vi "Calc Bearing Distance.vi"(10 "Current Location":cluster{"Latitude":ext, "Longitude":ext} {"Longitude" format="%#.6f"; "Latitude" format="%#.6f"}, 11 "Destination":cluster{"Latitude":ext, "Longitude":ext} {"Longitude" format="%#.6f"; "Latitude" format="%#.6f"}) -> (2 "Bearing to Destination":dbl, 3 "distance (m)":dbl)   [LabVIEW 2015, in "RDS Libraries.lvlib"]
uses:
  RDS Libraries.lvlib
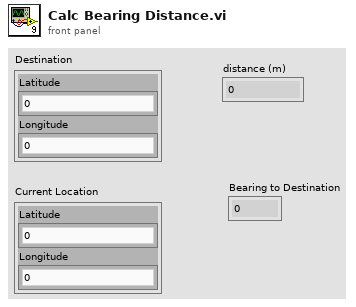
[diagram p1: front panel]
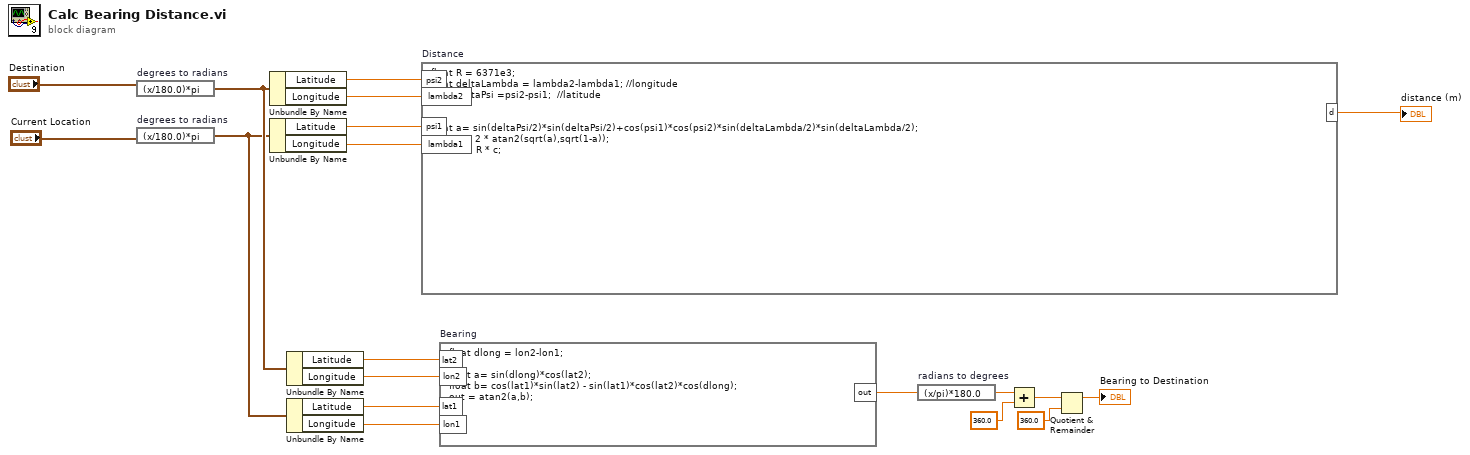
[diagram p0: block diagram]
diagram:
  n1 = expression code="(x/180.0)*pi" "degrees to radians"("Destination") -> (w4:cluster{"Latitude":ext, "Longitude":ext})
  n2 = expression code="(x/180.0)*pi" "degrees to radians"("Current Location") -> (w3:cluster{"Latitude":ext, "Longitude":ext})
  n3 = Unbundle By Name(w4) -> ("Latitude"=w17:ext, "Longitude"=w16:ext)
  n4 = Unbundle By Name(w3) -> ("Latitude"=w19:ext, "Longitude"=w18:ext)
  n5 = Unbundle By Name(w4) -> ("Latitude"=w12:ext, "Longitude"=w11:ext)
  n6 = Unbundle By Name(w3) -> ("Latitude"=w14:ext, "Longitude"=w13:ext)
  n7 = formula code="float R = 6371e3;\nfloat deltaLambda = lambda2-lambda1; //longitude\nfloat deltaPsi =psi2-psi1;  //latitude\n\n\nfloat a= sin(deltaPsi/2)*sin(deltaPsi/2)+cos(psi1)*cos(psi2)*sin(deltaLambda/2)*sin(deltaLambda/2);\nfloat c = 2 * atan2(sqrt(a),sqrt(1-a));\nfloat d = R * c;" "Distance"("psi1"=w19, "psi2"=w17, "lambda1"=w18, "lambda2"=w16) -> ("d"=→"distance (m)":dbl)
  n8 = formula code="float dlong = lon2-lon1;\n\nfloat a= sin(dlong)*cos(lat2);\nfloat b= cos(lat1)*sin(lat2) - sin(lat1)*cos(lat2)*cos(dlong);\nout = atan2(a,b);" "Bearing"("lat1"=w14, "lat2"=w12, "lon1"=w13, "lon2"=w11) -> ("out"=w10:dbl)
  n9 = expression code="(x/pi)*180.0" "radians to degrees"(w10) -> (w5:dbl)
  n10 = Add(x=w5, y=360.0) -> (x+y=w8:dbl)
  n11 = Quotient & Remainder(x=w8, y=360.0) -> (x-y*floor(x/y)=→"Bearing to Destination":dbl)  [unwired: 1 out]
